vi "Cancel State Machine.vi"(0 "What to Cancel":enum16{"Pickup", "Load"}(ring)) -> ()   [LabVIEW 2013]
uses:
  typedefs/subStates.ctl
  typedefs/fg_typedef.ctl
  typedefs/DevRef Type.ctl
  typedefs/singleUseSubstate.ctl
  <vilib>/Rock Robotics/WPI/Solenoid/WPI_SolenoidValue.ctl
  <vilib>/Rock Robotics/WPI/Solenoid/WPI_SolenoidGetEnum.vi
panel:
  # "A State Machine to Handle Canceling a Given Command"
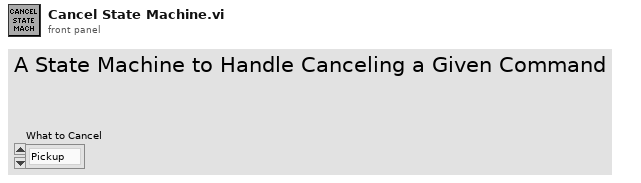
[diagram p1: front panel]
types:
  T1 = typedef "subStates.ctl" = enum16{"null", "wait", "driver control", "auto", "manual override", "hold position", "rotate", "pickup", "pass", "load", "goto shoot", "shoot high goal", "shoot low goal", "cancel arm", "cancel shooter", "end"}
  T2 = typedef "DevRef Type.ctl" = enum16{"Shooter Solenoid", "Latch Solenoid", "Right Up Sensor", "Right Down Sensor", "Hold Sensor", "2 Ball Switch", "Arm Encoder"}
  T3 = typedef "fg_typedef.ctl" = enum16{"Get", "Set"}
  T4 = typedef "WPI_SolenoidValue.ctl" = enum16{"Off", "On", "Forward", "Reverse"}
  T5 = typedef "singleUseSubstate.ctl" = enum16{"null", "wait", "shift high", "shift low", "extend shooter", "retract shooter", "latch", "unlatch", "end"}
  T6 = typedef "WPI_EncoderDevRef.ctl" = cluster{"DevStatus":errorcluster, "EncoderIndex":T7, "CounterIndex":T8, "DistancePerCount":dbl, "Decoding Type":T9}
  T7 = typedef "FPGA_EncoderIdx.ctl" = enum8{"Enc 0", "Enc 1", "Enc 2", "Enc 3", "Invalid"}
  T8 = typedef "FPGA_CounterCtrSystemIndex.ctl" = enum8{"Ctr 0", "Ctr 1", "Ctr 2", "Ctr 3", "Ctr 4", "Ctr 5", "Ctr 6", "Ctr 7", "Invalid"}
  T9 = typedef "WPI_EncoderType.ctl" = enum16{"1x", "2x", "4x"}
  T10 = typedef "WPI_DigitalInputDevRef.ctl" = cluster{"DevStatus":errorcluster, "DIO Channel":T11, "Digital Module":T12}
  T11 = typedef "FPGA_DIOChannel.ctl" = enum8{"DIO 1", "DIO 2", "DIO 3", "DIO 4", "DIO 5", "DIO 6", "DIO 7", "DIO 8", "DIO 9", "DIO 10", "DIO 11", "DIO 12", "DIO 13", "DIO 14", "Invalid"}
  T12 = typedef "FPGA_TypedefDigitalModule.ctl" = enum16{"Digital Module 1", "Digital Module 2"}
  T13 = typedef "WPI_SolenoidDevRef.ctl" = cluster{"DevStatus":errorcluster, "Solenoid Module":T14, "Forward Solenoid Channel":T15, "Reverse Solenoid Channel":T15}
  T14 = typedef "FPGA_TypedefSolenoidModule.ctl" = enum16{"Solenoid Module 1", "Solenoid Module 2"}
  T15 = typedef "WPI_SolenoidChannel.ctl" = enum8{"Solenoid 1", "Solenoid 2", "Solenoid 3", "Solenoid 4", "Solenoid 5", "Solenoid 6", "Solenoid 7", "Solenoid 8", "Invalid"}
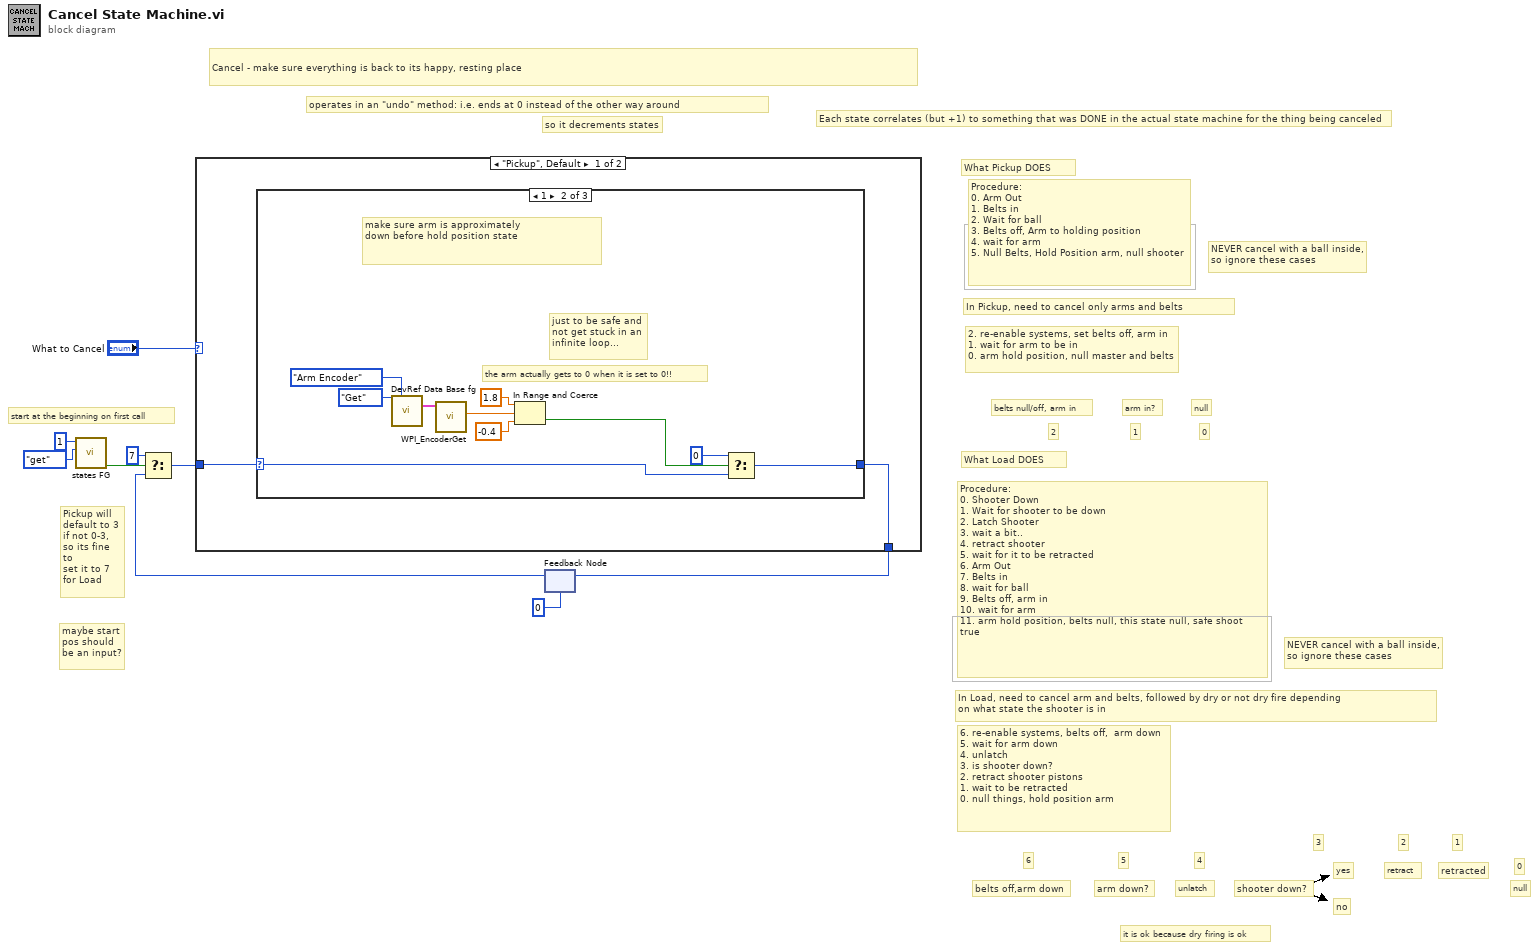
[diagram p0: block diagram]
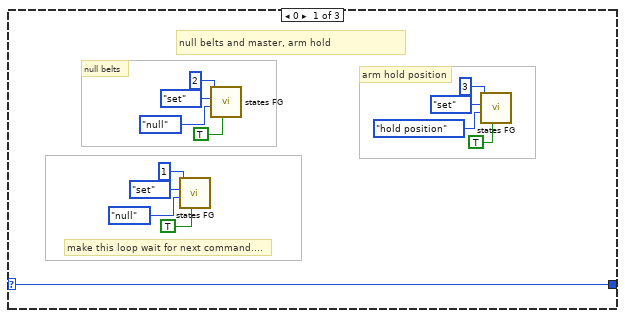
[diagram p2: hidden frame]
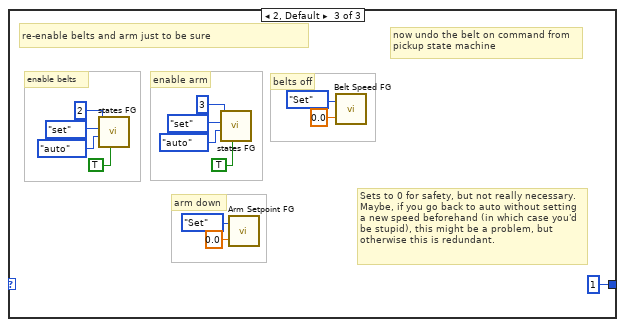
[diagram p3: hidden frame]
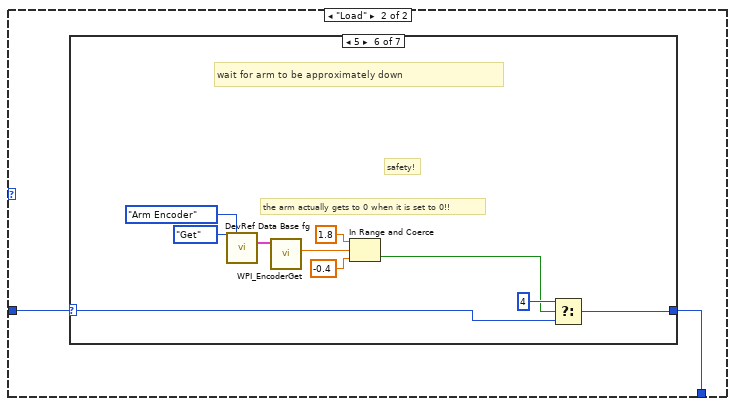
[diagram p4: hidden frame]
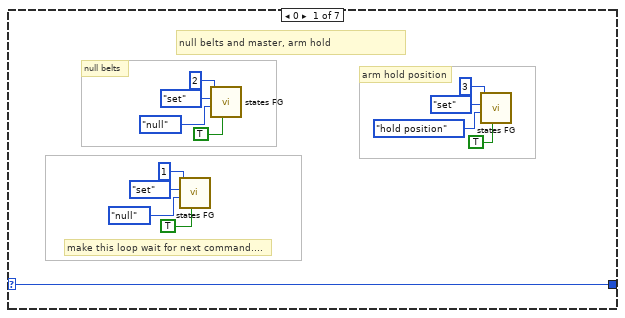
[diagram p5: hidden frame]
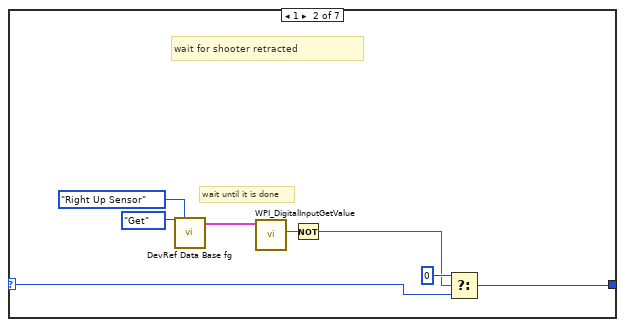
[diagram p6: hidden frame]
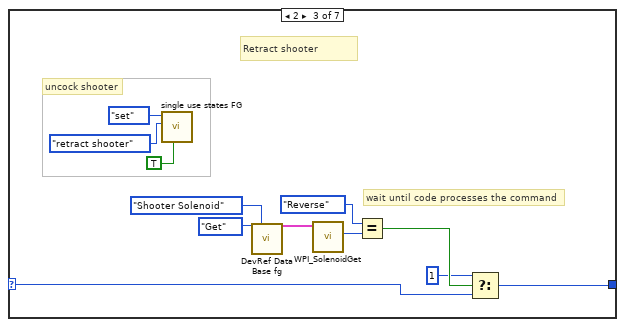
[diagram p7: hidden frame]
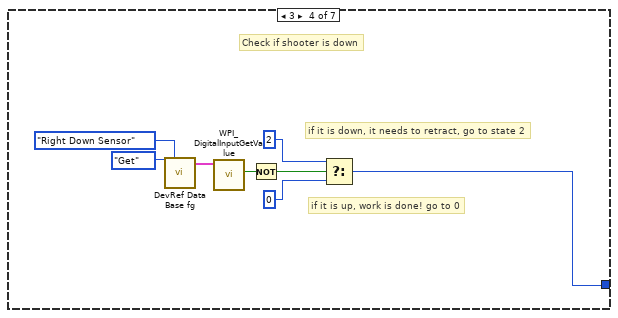
[diagram p8: hidden frame]
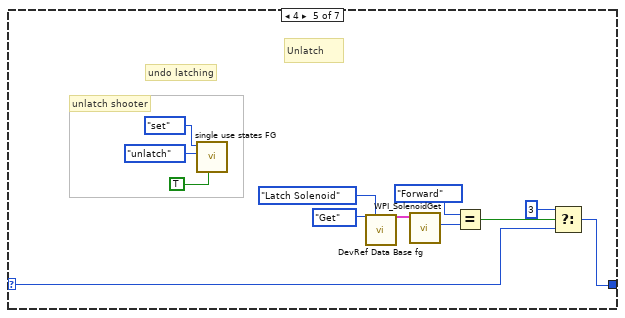
[diagram p9: hidden frame]
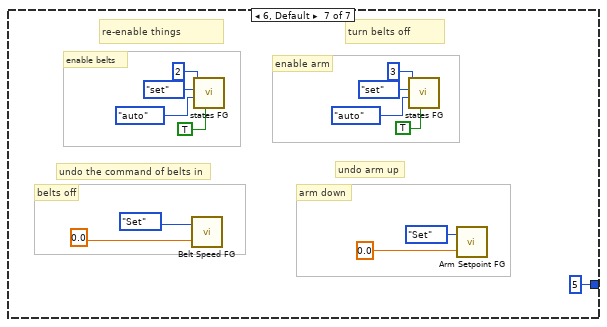
[diagram p10: hidden frame]
diagram:
  # "maybe start\npos should\nbe an input?"
  # "Pickup will\ndefault to 3\nif not 0-3,\nso its fine to\nset it to 7\nfor Load"
  # "1"
  # "retracted"
  # "5"
  # "arm down?"
  # "it is ok because dry firing is ok"
  # "Procedure: \n0. Shooter Down \n1. Wait for shooter to be down\n2. Latch Shooter\n3. wait a bit..\n4. retract shooter\n5. wait for it to be retracted\n6. Arm Out\n7. Belts in\n8. wait for ball\n9. Belts off, arm in\n10. wait for arm\n11. arm hold position, belts null, this state null, safe shoot true"
  # "0"
  # "null"
  # "1"
  # "2"
  # "arm in?"
  # "belts null/off, arm in"
  # "0"
  # "2"
  # "3"
  # "4"
  # "6"
  # "null"
  # "unlatch"
  # "retract"
  # "no"
  # "yes"
  # "shooter down?"
  # "belts off,arm down"
  # "NEVER cancel with a ball inside,\nso ignore these cases"
  # "What Load DOES"
  # "NEVER cancel with a ball inside,\nso ignore these cases"
  # "so it decrements states"
  # "What Pickup DOES"
  # "Each state correlates (but +1) to something that was DONE in the actual state machine for the thing being canceled"
  # "6. re-enable systems, belts off,  arm down\n5. wait for arm down\n4. unlatch\n3. is shooter down?\n2. retract shooter pistons\n1. wait to be retracted\n0. null things, hold position arm"
  # "In Load, need to cancel arm and belts, followed by dry or not dry fire depending\non what state the shooter is in"
  # "operates in an \"undo\" method: i.e. ends at 0 instead of the other way around"
  # "2. re-enable systems, set belts off, arm in\n1. wait for arm to be in\n0. arm hold position, null master and belts"
  # "In Pickup, need to cancel only arms and belts"
  # "start at the beginning on first call"
  # "Cancel - make sure everything is back to its happy, resting place"
  # "Procedure: \n0. Arm Out\n1. Belts in\n2. Wait for ball\n3. Belts off, Arm to holding position\n4. wait for arm\n5. Null Belts, Hold Position arm, null shooter"
  n1 = call "states FG.vi"("menu (get)"=enum16{"set", "get"}."get", "Loop ID"=1) -> ("first call?"=w9:bool)  [unwired: 6 in, 3 out]
  n2 = feedback #1(u8 0) -> (w4:u8)
  n3 = Select(t=u8 7, s=w9, f=w4) -> (s? t:f=w6:u8)
  n4 = case shown="\"Pickup\", Default" "What to Cancel" {
    tunnel: w6 -> [w11 w49]
    tunnel: [w10 w48] -> w3
    frame "Pickup", Default {
      n5 = case shown="1" w11 {
        selector: w11 -> [w24 w28 _]
        tunnel: [w24 w27 u8 1 ("t")] -> w10
        frame 0 {
          # "null belts and master, arm hold"
          # "make this loop wait for next command...."
          # "arm hold position"
          # "null belts"
          n6 = call "states FG.vi"("exit in"=TRUE, "subState in"=subStates."null", "menu (get)"=enum16{"set", "get"}."set", "Loop ID"=1) -> ()  [unwired: 4 in, 4 out]
          n7 = call "states FG.vi"("exit in"=TRUE, "subState in"=subStates."null", "menu (get)"=enum16{"set", "get"}."set", "Loop ID"=2) -> ()  [unwired: 4 in, 4 out]
          n8 = call "states FG.vi"("exit in"=TRUE, "subState in"=subStates."hold position", "menu (get)"=enum16{"set", "get"}."set", "Loop ID"=3) -> ()  [unwired: 4 in, 4 out]
        }
        frame 1 {
          # "just to be safe and\nnot get stuck in an \ninfinite loop..."
          # "the arm actually gets to 0 when it is set to 0!!"
          # "make sure arm is approximately\ndown before hold position state"
          n9 = call "DevRef Data Base fg.vi"("Menu"=fg_typedef."Get", "DevRef to Get"=DevRef_Type."Arm Encoder") -> ("Selected Encoder"=w32:T6)  [unwired: 23 in, 2 out]
          n10 = call <vilib>:"WPI_EncoderGet.vi"("EncoderDevRef"=w32) -> ("Distance"=w31:dbl)  [unwired: 5 in, 5 out]
          n11 = In Range and Coerce(upper limit=1.8, x=w31, lower limit=-0.4 ("upper limit")) -> (In Range?=w25:bool)  [unwired: 1 out]
          n12 = Select(t=u8 0, s=w25, f=w28) -> (s? t:f=w27:u8)
        }
        frame 2, Default {
          # "arm down"
          # "Sets to 0 for safety, but not really necessary.\nMaybe, if you go back to auto without setting\na new speed beforehand (in which case you'd\nbe stupid), this might be a problem, but\notherwise this is redundant."
          # "now undo the belt on command from\npickup state machine"
          # "belts off"
          # "re-enable belts and arm just to be sure"
          # "enable arm"
          # "enable belts"
          n13 = call "states FG.vi"("exit in"=TRUE, "subState in"=subStates."auto", "menu (get)"=enum16{"set", "get"}."set", "Loop ID"=2) -> ()  [unwired: 4 in, 4 out]
          n14 = call "states FG.vi"("exit in"=TRUE, "subState in"=subStates."auto", "menu (get)"=enum16{"set", "get"}."set", "Loop ID"=3) -> ()  [unwired: 4 in, 4 out]
          n15 = call "Arm Setpoint FG.vi"("Setpoint In"=0.0, "Menu"=fg_typedef."Set") -> ()  [unwired: 1 out]
          n16 = call "Belt Speed FG.vi"("Speed In"=0.0 ("Setpoint In"), "Menu"=fg_typedef."Set") -> ()  [unwired: 1 out]
        }
      }
    }
    frame "Load" {
      n17 = case shown="5" w49 {
        selector: w49 -> [w62 w66 w79 _ w94 w106 _]
        tunnel: [w62 w65 w78 w86 w93 w105 u8 5 ("t")] -> w48
        frame 0 {
          # "null belts and master, arm hold"
          # "make this loop wait for next command...."
          # "arm hold position"
          # "null belts"
          n18 = call "states FG.vi"("exit in"=TRUE, "subState in"=subStates."null", "menu (get)"=enum16{"set", "get"}."set", "Loop ID"=1) -> ()  [unwired: 4 in, 4 out]
          n19 = call "states FG.vi"("exit in"=TRUE, "subState in"=subStates."null", "menu (get)"=enum16{"set", "get"}."set", "Loop ID"=2) -> ()  [unwired: 4 in, 4 out]
          n20 = call "states FG.vi"("exit in"=TRUE, "subState in"=subStates."hold position", "menu (get)"=enum16{"set", "get"}."set", "Loop ID"=3) -> ()  [unwired: 4 in, 4 out]
        }
        frame 1 {
          # "wait until it is done"
          # "wait for shooter retracted"
          n21 = call "DevRef Data Base fg.vi"("Menu"=fg_typedef."Get", "DevRef to Get"=DevRef_Type."Right Up Sensor") -> ("Selected Sensor"=w68:T10)  [unwired: 23 in, 2 out]
          n22 = call <vilib>:"WPI_DigitalInputGetValue.vi"("DigitalInputDevRef"=w68) -> ("Value"=w70:bool)  [unwired: 8 in, 2 out]
          n23 = Not(x=w70) -> (.not. x?=w63:bool)
          n24 = Select(t=u8 0, s=w63, f=w66) -> (s? t:f=w65:u8)
        }
        frame 2 {
          # "wait until code processes the command"
          # "uncock shooter"
          # "Retract shooter"
          n25 = call "single use states FG.vi"("exit in"=TRUE, "substate"=singleUseSubstate."retract shooter", "menu (get)"=enum16{"set", "get"}."set") -> ()  [unwired: 5 in, 4 out]
          n26 = call "DevRef Data Base fg.vi"("Menu"=fg_typedef."Get", "DevRef to Get"=DevRef_Type."Shooter Solenoid") -> ("Selected Solenoid"=w75:T13)  [unwired: 23 in, 2 out]
          n27 = call-poly <vilib>:"WPI_SolenoidGet.vi"("SolenoidDevRef"=w75) -> ("Value"=w74:T4)  [unwired: 8 in, 2 out]
          n28 = Equal?(x=WPI_SolenoidValue."Reverse", y=w74) -> (x = y?=w72:bool)
          n29 = Select(t=u8 1, s=w72, f=w79) -> (s? t:f=w78:u8)
        }
        frame 3 {
          # "if it is up, work is done! go to 0"
          # "if it is down, it needs to retract, go to state 2"
          # "Check if shooter is down"
          n30 = call "DevRef Data Base fg.vi"("Menu"=fg_typedef."Get", "DevRef to Get"=DevRef_Type."Right Down Sensor") -> ("Selected Sensor"=w88:T10)  [unwired: 23 in, 2 out]
          n31 = call <vilib>:"WPI_DigitalInputGetValue.vi"("DigitalInputDevRef"=w88) -> ("Value"=w89:bool)  [unwired: 8 in, 2 out]
          n32 = Not(x=w89) -> (.not. x?=w87:bool)
          n33 = Select(t=u8 2, s=w87, f=u8 0) -> (s? t:f=w86:u8)
        }
        frame 4 {
          # "unlatch shooter"
          # "undo latching"
          # "Unlatch"
          n34 = call "single use states FG.vi"("exit in"=TRUE, "substate"=singleUseSubstate."unlatch", "menu (get)"=enum16{"set", "get"}."set") -> ()  [unwired: 5 in, 4 out]
          n35 = call "DevRef Data Base fg.vi"("Menu"=fg_typedef."Get", "DevRef to Get"=DevRef_Type."Latch Solenoid") -> ("Selected Solenoid"=w98:T13)  [unwired: 23 in, 2 out]
          n36 = call-poly <vilib>:"WPI_SolenoidGet.vi"("SolenoidDevRef"=w98) -> ("Value"=w96:T4)  [unwired: 8 in, 2 out]
          n37 = Equal?(x=WPI_SolenoidValue."Forward" ("Value"), y=w96) -> (x = y?=w95:bool)
          n38 = Select(t=u8 3, s=w95, f=w94) -> (s? t:f=w93:u8)
        }
        frame 5 {
          # "safety!"
          # "wait for arm to be approximately down"
          # "the arm actually gets to 0 when it is set to 0!!"
          n39 = call "DevRef Data Base fg.vi"("Menu"=fg_typedef."Get", "DevRef to Get"=DevRef_Type."Arm Encoder") -> ("Selected Encoder"=w110:T6)  [unwired: 23 in, 2 out]
          n40 = call <vilib>:"WPI_EncoderGet.vi"("EncoderDevRef"=w110) -> ("Distance"=w109:dbl)  [unwired: 5 in, 5 out]
          n41 = In Range and Coerce(upper limit=1.8, x=w109, lower limit=-0.4 ("upper limit")) -> (In Range?=w103:bool)  [unwired: 1 out]
          n42 = Select(t=u8 4, s=w103, f=w106) -> (s? t:f=w105:u8)
        }
        frame 6, Default {
          # "undo arm up"
          # "arm down"
          # "re-enable things"
          # "turn belts off"
          # "undo the command of belts in"
          # "belts off"
          # "enable arm"
          # "enable belts"
          n43 = call "Belt Speed FG.vi"("Speed In"=0.0 ("Setpoint In"), "Menu"=fg_typedef."Set") -> ()  [unwired: 1 out]
          n44 = call "states FG.vi"("exit in"=TRUE, "subState in"=subStates."auto", "menu (get)"=enum16{"set", "get"}."set", "Loop ID"=2) -> ()  [unwired: 4 in, 4 out]
          n45 = call "states FG.vi"("exit in"=TRUE, "subState in"=subStates."auto", "menu (get)"=enum16{"set", "get"}."set", "Loop ID"=3) -> ()  [unwired: 4 in, 4 out]
          n46 = call "Arm Setpoint FG.vi"("Setpoint In"=0.0, "Menu"=fg_typedef."Set") -> ()  [unwired: 1 out]
        }
      }
    }
  }
  n47 = feedback-in #1(w3) -> ()
